vi "Hide Loader.vi"(8 "error in (no error)":errorcluster, 11 "VI in":refnum<vi>) -> (0 "error out":errorcluster)   [LabVIEW 2019, in "gRPC Template Creation Utility.lvlib"]
uses:
  gRPC Template Creation Utility.lvlib
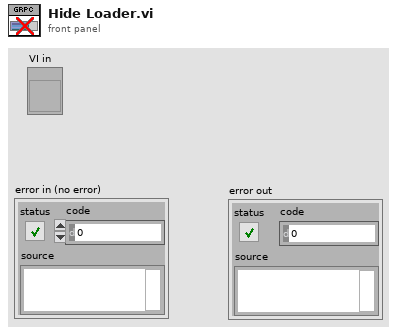
[diagram p1: front panel]
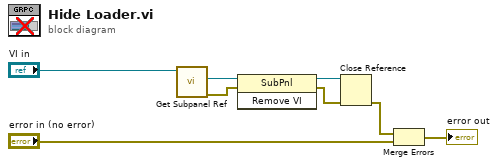
[diagram p0: block diagram]
diagram:
  n1 = call "Get Subpanel Ref.vi"("Owner VI in"="VI in") -> ("error out"=w4:errorcluster, "SubPanel out"=w7:refnum<vi>)  [unwired: 9 in]
  n2 = invoke class="SubPnl" method="Remove VI"(reference=w7, error in=w4) -> (reference out=w5:refnum<vi>, error out=w6:errorcluster)  [unwired: 1 in, 1 out]
  n3 = Close Reference(reference=w5, error in (no error)=w6) -> (error out=w2:errorcluster)
  n4 = Merge Errors(w2, "error in (no error)") -> (→"error out":errorcluster)
